vi "VIremote_VIs_for_BELLA.vi"(8 "error in (no error)":errorcluster) -> (0 "error out":errorcluster, 3 "Strings []":string[](array[string]))   [LabVIEW 2013]
panel:
  in  "Listbox to change order (drag)":i32(listbox)=8
  # "Bella_M1Cam_GUI-viremote.vi"
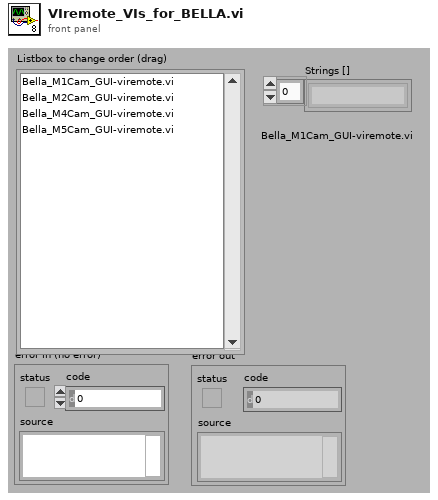
[diagram p1: front panel]
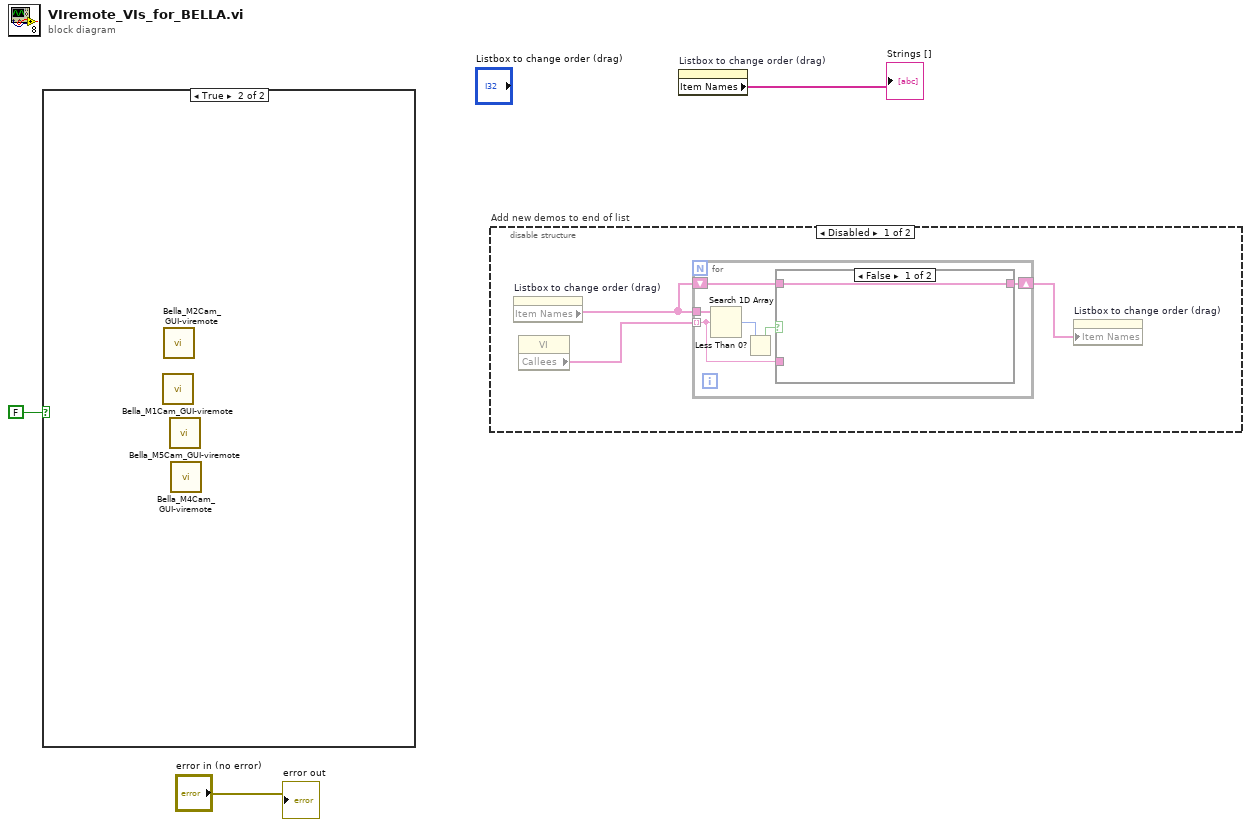
[diagram p0: block diagram]
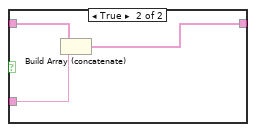
[diagram p2: hidden frame]
diagram:
  n1 = case shown="True" FALSE {
    frame False {
    }
    frame True {
      n2 = call "Bella_M1Cam_GUI-viremote.vi"() -> ()  [unwired: 11 in, 1 out]
      n3 = call "Bella_M2Cam_GUI-viremote.vi"() -> ()  [unwired: 11 in, 1 out]
      n4 = call "Bella_M5Cam_GUI-viremote.vi"() -> ()  [unwired: 11 in, 1 out]
      n5 = call "Bella_M4Cam_GUI-viremote.vi"() -> ()  [unwired: 11 in, 1 out]
    }
  }
  n6 = disable-structure "Add new demos to end of list" shown="Disabled" {
    frame Disabled {
      n7 = property on="Listbox to change order (drag)" class="LstBox (strict)"() -> ("Item Names"=w5:string[])  [unwired: 2 in, 2 out]
      n8 = property class="VI"() -> ("Callees"=w6:string[])  [unwired: 2 in, 2 out]
      n9 = for {
        tunnel: w5 -> [w12]
        tunnel: w6 -> [w8] mode=indexing
        shift-right: [w7] -> w4
        shift-left: w5 -> [w9]
        n10 = Search 1D Array(1D array=w12, element=w8) -> (index of element=w11:i32)  [unwired: 1 in]
        n11 = Less Than 0?(x=w11) -> (x < 0?=w10:bool)
        n12 = case shown="False" w10 {
          tunnel: w9 -> [w13 w16]
          tunnel: w8 -> [_ w15]
          tunnel: [w13 w14] -> w7
          frame False {
          }
          frame True {
            n13 = Build Array (concatenate)(w16, w15) -> (w14:string[])
          }
        }
      }
      n14 = property on="Listbox to change order (drag)" class="LstBox (strict)"("Item Names"=w4) -> ()  [unwired: 2 in, 2 out]
    }
    frame Enabled {
    }
  }
  n15 = property on="Listbox to change order (drag)" class="LstBox (strict)"() -> ("Item Names"=→"Strings []":string[])  [unwired: 2 in, 2 out]
  "error out" <- "error in (no error)"
